vi "Dev - Filter List Module.vi"(8 "Error In":errorcluster, 11 "Module In":string[](array[string])) -> (0 "Error Out":errorcluster, 2 "RT Module":string[](array[string]), 3 "HMI Module":string[](array[string]))   [LabVIEW 2020]
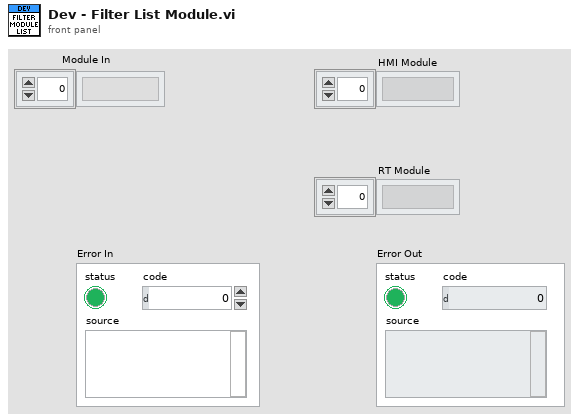
[diagram p1: front panel]
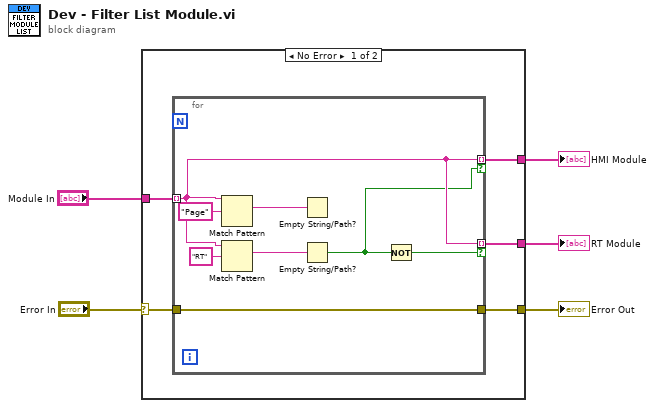
[diagram p0: block diagram]
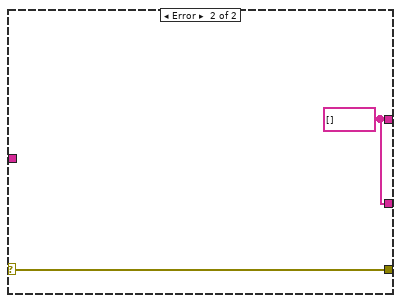
[diagram p2: hidden frame]
diagram:
  n1 = case shown="No Error" "Error In" {
    selector: "Error In" -> [w9 w20]
    tunnel: [w10 w20] -> w4
    tunnel: "Module In" -> [w8 _]
    tunnel: [w7 w19] -> w2
    tunnel: [w6 w19] -> w1
    frame No Error {
      n2 = for {
        tunnel: w8 -> [w15] mode=indexing
        tunnel: [w18] -> w10
        tunnel: w9 -> [w18]
        tunnel: [w15] -> w7 mode=indexing if=w11
        tunnel: [w15] -> w6 mode=indexing if=w12
        n3 = Match Pattern(string=w15, regular expression="Page") -> (match substring=w17:string)  [unwired: 1 in, 3 out]
        n4 = Match Pattern(string=w15, regular expression="RT") -> (match substring=w13:string)  [unwired: 1 in, 3 out]
        n5 = Empty String/Path?(string/path=w17) -> ()  [unwired: 1 out]
        n6 = Empty String/Path?(string/path=w13) -> (empty?=w11:bool)
        n7 = Not(x=w11) -> (.not. x?=w12:bool)
      }
    }
    frame Error {
      w19 = string[] []
    }
  }
  "Error Out" <- w4
  "HMI Module" <- w2
  "RT Module" <- w1
